vi "RSZVB Get Calibration Power Offset.vi"(8 "error in (no error)":errorcluster {"code" format="%.0x"}, 9 "Port Number (1)":i32=1, 10 "Channel (1)":i32=1, 11 "VISA session":refnum<visa-resource-name>) -> (0 "error out":errorcluster {"code" format="%.0x"}, 2 "Calibration Power Offset":dbl format="%^.3e", 3 "dup VISA session":refnum<visa-resource-name>)   [LabVIEW 2011]
doc: "This VI returns a gain (positive values) or an attenuation (negative values) in the signal path between the source port and the calibrated reference plane.\n\nRemote-control command(s):\nSOURce<Ch>:POWer<Pt>:CORRection:LEVel:OFFSet?"
uses:
  _utility/RSZVB Global Data.vi
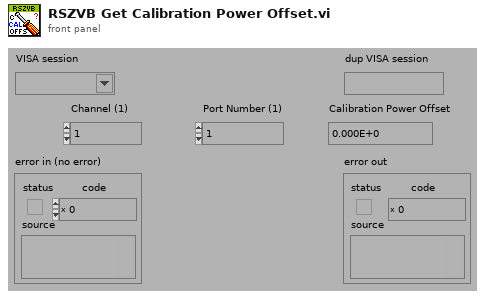
[diagram p1: front panel]
types:
  T1 = cluster{"Error Checking (T: On)":bool, "Installed Options":string[], "Data Valid?":bool, "Ports":i32, "Model":string[], "Option Checking (T: On)":bool}[]
  T2 = cluster{"Error Checking (T: On)":bool, "Installed Options":string[], "Data Valid?":bool, "Ports":i32, "Model":string[], "Option Checking (T: On)":bool}
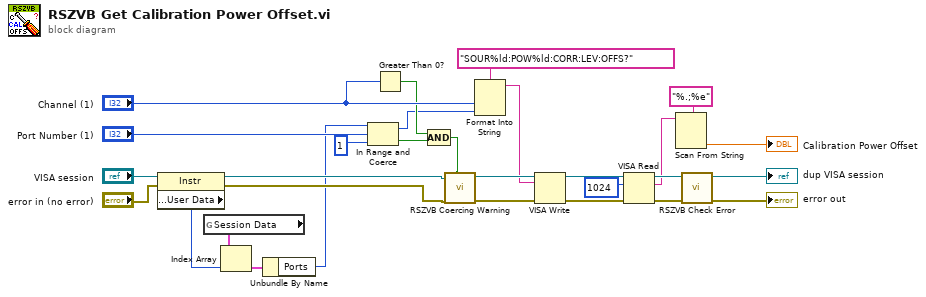
[diagram p0: block diagram]
diagram:
  n1 = property class="Instr"(reference="VISA session", error in="error in (no error)") -> (reference out=w9:refnum<visa-resource-name>, error out=w8:errorcluster, "General Settings:User Data"=w10:u32)
  n2 = global read "RSZVB Global Data.vi" "Session Data"() -> (w11:T1)
  n3 = Index Array(array=w11, index=w10) -> (element=w12:T2)
  n4 = Unbundle By Name(w12) -> ("Ports"=w1:i32)
  n5 = In Range and Coerce(upper limit=w1, x="Port Number (1)", lower limit=1) -> (coerced(x)=w2:i32, In Range?=w3:bool)
  n6 = Greater Than 0?(x="Channel (1)") -> (x > 0?=w14:bool)
  n7 = Compound Arithmetic op=AND(w14, w3) -> (w13:bool)
  n8 = call "RSZVB Coercing Warning.vi"("In Range?"=w13, "error in (no error)"=w8, "VISA session"=w9) -> ("error out"=w21:errorcluster, "dup VISA session"=w22:refnum<visa-resource-name>)  [unwired: 7 in]
  n9 = Format Into String(format string="SOUR%ld:POW%ld:CORR:LEV:OFFS?", "Channel (1)", w2) -> (resulting string=w19:string)  [unwired: 2 in, 1 out]
  n10 = VISA Write(VISA resource name=w22, write buffer=w19, error in (no error)=w21) -> (VISA resource name out=w23:refnum<visa-resource-name>, error out=w24:errorcluster)  [unwired: 1 out]
  n11 = VISA Read(VISA resource name=w23, byte count=u32 1024 ("byte count (0)"), error in (no error)=w24) -> (VISA resource name out=w28:refnum<visa-resource-name>, read buffer=w25:string, error out=w27:errorcluster)  [unwired: 1 out]
  n12 = Scan From String(format string="%.;%e", input string=w25) -> (output 1=→"Calibration Power Offset":dbl)  [unwired: 3 in, 3 out]
  n13 = call "RSZVB Check Error.vi"("error in (no error)"=w27, "VISA session"=w28) -> ("error out"=→"error out":errorcluster, "dup VISA session"=→"dup VISA session":refnum<visa-resource-name>)  [unwired: 8 in]
